vi "DI IRQ Config Pane.vi"(6 "_SubPanelMessages":refnum<notifier>, 9 "_myEmbeddedToFrameEvent":T7, 10 "_myEmbedded.Exit":refnum<user-event>, 11 "_Property Bundle":cluster{"Name":string, "Value":variant}[](array[cluster])) -> (1 "_Connection Informations":T2, 2 "_Scripter Input":T4)   [LabVIEW 2021]
doc: "Registers analog and digital input interrupts and creates timer interrupts."
uses:
  <vilib>/myRIO/Common/Express VI Framework/xctls/myRIO Channel Name/myRIO Channel Name.xctl
  <vilib>/myRIO/Common/Instrument Driver Framework/myRIO v1.0/IRQ/typedefs/DI IRQ Type.ctl
  <vilib>/myRIO/Common/Express VI Framework/typedefs/Config Pane to Framework Ref.ctl
  <vilib>/myRIO/Common/Express VI Framework/typedefs/Data Validate Ref.ctl
  <vilib>/myRIO/Common/Express VI Framework/typedefs/Sub Panel Messages.ctl
  <vilib>/myRIO/Common/Express VI Framework/typedefs/Instrument Driver Method Descriptor Array.ctl
  <vilib>/myRIO/Common/Express VI Framework/typedefs/Instrument Driver Method Descriptor.ctl
  <vilib>/myRIO/Common/Express VI Framework/typedefs/Scripter Input.ctl
  <vilib>/myRIO/Common/Express VI Framework/typedefs/WireThrough Terminal Names.ctl
  <vilib>/myRIO/Common/Express VI Framework/typedefs/Connection Informations.ctl
  <vilib>/myRIO/Common/Instrument Driver Framework/Utilities/typedefs/Channel Types.ctl
  <vilib>/myRIO/Common/Express VI Framework/vis/Express VI Framework Strings Global.vi
  <vilib>/myRIO/Express VI/IRQ/Message Globals.vi
panel:
  out "_create Callback?":bool
  in  "_Create Button":bool
  in  "Callback VI Path:":path
  out "_Warning Icon":picture
  out "_Callback VI Path":string caption="Callback VI:"
  in  "_Open Button":bool
  out "_Count Label":string
  out "_Counts":string[](array[string])=["", "1", "", "1", "", "1", "", "1", "", "1", "", "1"]
  out "_Digtal Preview":T1(graph) caption="Preview:"
  out "_Error Message":string
  in  "_callback":refnum<vi>
  in  "_VI Default Name (Edit and make value default)":string="Digital input interrupt"
  in  "_WireThrough Info (Edit and make value default)":T3={"WireThrough Top In"="Ref In", "WireThrough Bottom In"="error in (no error)", "WireThrough Top Out"="Ref Out", "WireThrough Bottom Out"="error out"}
  in  "_Template Array (Edit and make value default)":T5=[{"Function Name"="Register DI IRQ", "VI Path"=path "<vilib>/myRIO/Instrument Drivers/IRQ/IO IRQ/vis", "Script"=TRUE, "Inputs"=[{"name"="IRQ Number", "value"=variant, "Config Pane Only"=TRUE, "Build Array"=FALSE, "Bundle Cluster"=FALSE, "Show Term"=FALSE, "alias"=[], "Required Input"=FALSE}, {"name"="Digital Interrupt Type", "value"=variant, "Config Pane Only"=TRUE, "Build Array"=FALSE, "Bundle Cluster"=FALSE, "Show Term"=FALSE, "alias"=[], "Required Input"=FALSE}, {"name"="Channel Name", "value"=variant, "Config Pane Only"=TRUE, "Build Array"=FALSE, "Bundle Cluster"=FALSE, "Show Term"=FALSE, "alias"=[], "Required Input"=FALSE}, {"name"="Edge Count", "value"=variant, "Config Pane Only"=TRUE, "Build Array"=FALSE, "Bundle Cluster"=FALSE, "Show Term"=FALSE, "alias"=[], "Required Input"=FALSE}, {"name"="Callback VI Reference", "value"=variant, "Config Pane Only"=FALSE, "Build Array"=FALSE, "Bundle Cluster"=FALSE, "Show Term"=TRUE, "alias"=[], "Required Input"=FALSE}], "Outputs"=[], "VI Class"=enum."Open", "Controls Refs[]"=[], "Inline"=FALSE}]
  in  "_Default Alias String":string
  in  "Type:":T9
  in  "Channel:":u16(xcontrol)
  in  "IRQ number:":u8 max=7
  in  "Edge count:":u32=1 min=1
  in  "Name:":string="Digital input interrupt" caption="Node name:"
  out "_IRQ Learn More":string="Interrupt triggers every time the number of edges reaches the specified Edge count. "
  # "NOTE: Tab Order has been set\nfor this Front Panel.\n\nSee Edit>>Set Tabbing Order...\n\nAll controls that are not visible at \nruntime are excluded from Tabbing order\n\nTo exlude a control from context\nhelp prefix its label text with a '-'"
  # "Trigger point"
  # "Digital input"
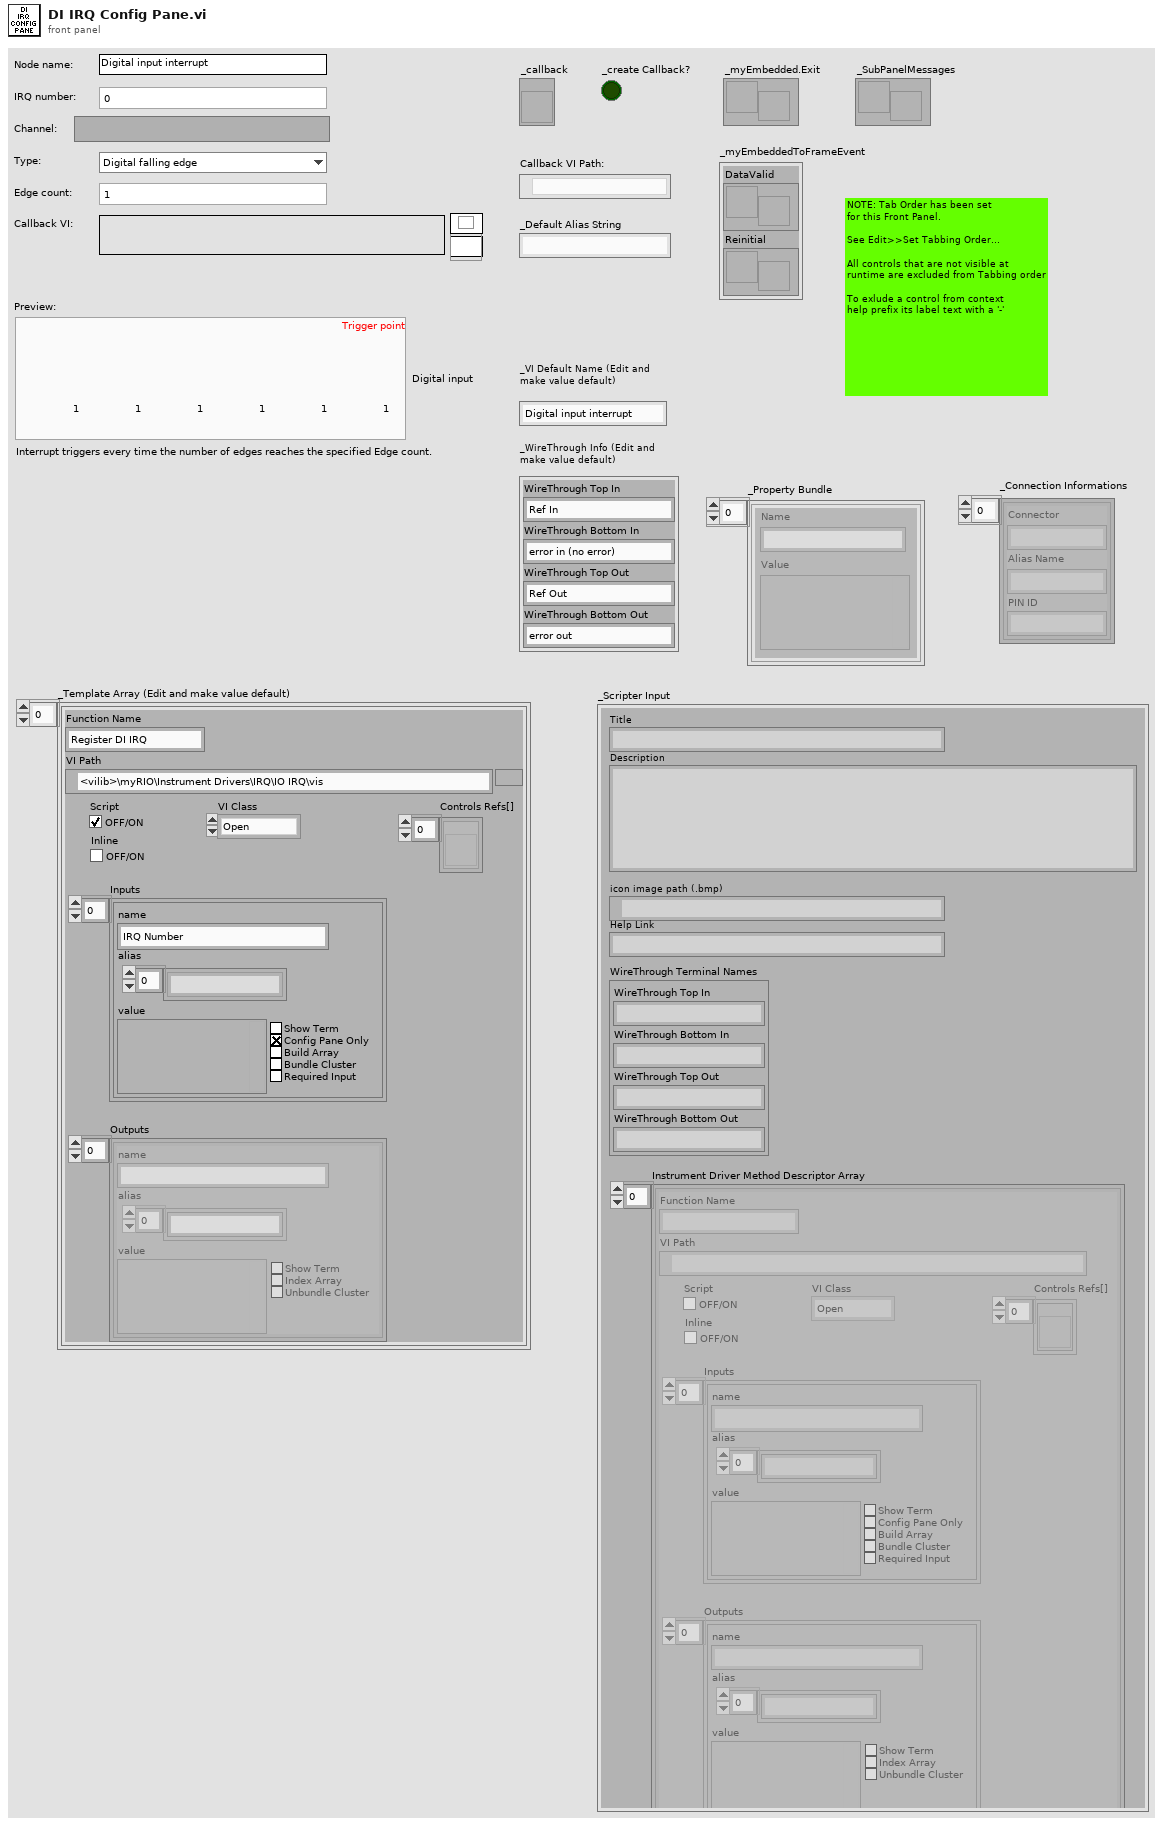
[diagram p1: front panel]
types:
  T1 = cluster{"Analog Preview 3":cluster{"X":dbl, "Y":dbl}[]}[]
  T2 = typedef "Connection Informations.ctl" = cluster{"Connector":string, "Alias Name":string, "PIN ID":string}[]
  T3 = typedef "WireThrough Terminal Names.ctl" = cluster{"WireThrough Top In":string, "WireThrough Bottom In":string, "WireThrough Top Out":string, "WireThrough Bottom Out":string}
  T4 = typedef "Scripter Input.ctl" = cluster{"Title":string, "Description":string, "icon image path (.bmp)":path, "Help Link":string, "WireThrough Terminal Names":T3, "Instrument Driver Method Descriptor Array":T5}
  T5 = typedef "Instrument Driver Method Descriptor Array.ctl" = T6[]
  T6 = typedef "Instrument Driver Method Descriptor.ctl" = cluster{"Function Name":string, "VI Path":path, "Script":bool, "Inputs":cluster{"name":string, "value":variant, "Config Pane Only":bool, "Build Array":bool, "Bundle Cluster":bool, "Show Term":bool, "alias":string[], "Required Input":bool}[], "Outputs":cluster{"name":string, "value":variant, "Show Term":bool, "Index Array":bool, "Unbundle Cluster":bool, "alias":string[]}[], "VI Class":enum16{"Open", "Configure", "Data", "Manage", "Close"}, "Controls Refs[]":refnum<vi>[], "Inline":bool}
  T7 = typedef "Config Pane to Framework Ref.ctl" = cluster{"DataValid":T8, "Reinitial":refnum<user-event>}
  T8 = typedef "Data Validate Ref.ctl" = refnum<user-event>
  T9 = typedef "DI IRQ Type.ctl" = enum16{"Digital falling edge", "Digital rising edge", "Digital edge"}
  T10 = typedef "Channel Types.ctl" = enum32{"Unknown", "AI", "AO", "DIO - DI", "DIO", "DIO - DO", "I2C", "PWM", "Encoder", "SPI", "UART", "Accelerometer", "DIO - LED", "DIO - Button", "AI (N Samples)", "AudioIn (N Samples)", "AO (N Samples)", "AudioOut (N Samples)", "DI (N Samples)", "DO (N Samples)", "AI IRQ", "DI IRQ", "Timer IRQ", "RSL", "Relay", "CAN", "AI (Continuous)", "AO (Continuous)"}
  T11 = typedef "Channel Info.ctl" = cluster{"Channel Name":string, "Alias":string, "Used?":bool, "Not Support?":bool, "Property Bundle":cluster{"Name":string, "Value":variant}[]}
  T12 = typedef "Sub Panel Messages.ctl" = enum16{"Initialized"}
  T13 = cluster{"Connector":string, "Alias Name":string, "PIN ID":string}
  T14 = cluster{"left":i16, "top":i16, "right":i16, "bottom":i16}
  T15 = cluster{"name":string, "value":variant, "Config Pane Only":bool, "Build Array":bool, "Bundle Cluster":bool, "Show Term":bool, "alias":string[], "Required Input":bool}[]
  T16 = cluster{"name":string, "value":variant, "Config Pane Only":bool, "Build Array":bool, "Bundle Cluster":bool, "Show Term":bool, "alias":string[], "Required Input":bool}
  T17 = cluster{"Connector":string, "Alias Name":string, "PIN ID":string}[]
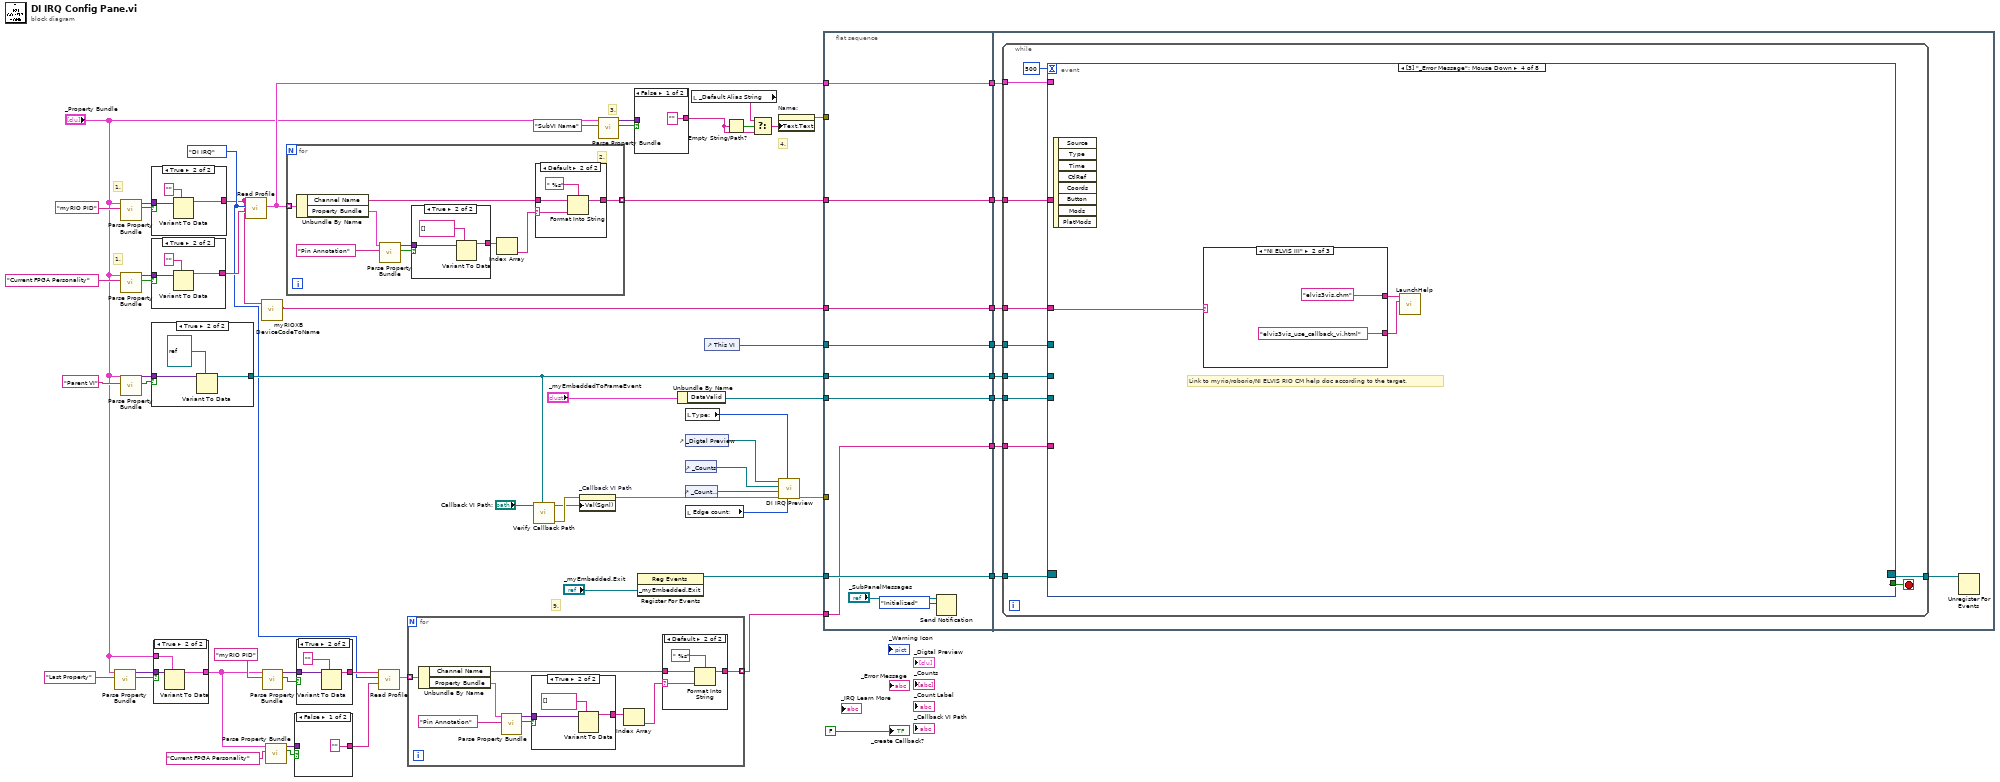
[diagram p0: block diagram]
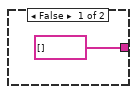
[diagram p2: hidden frame]
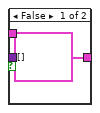
[diagram p4: hidden frame]
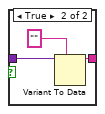
[diagram p5: hidden frame]
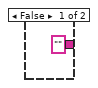
[diagram p6: hidden frame]
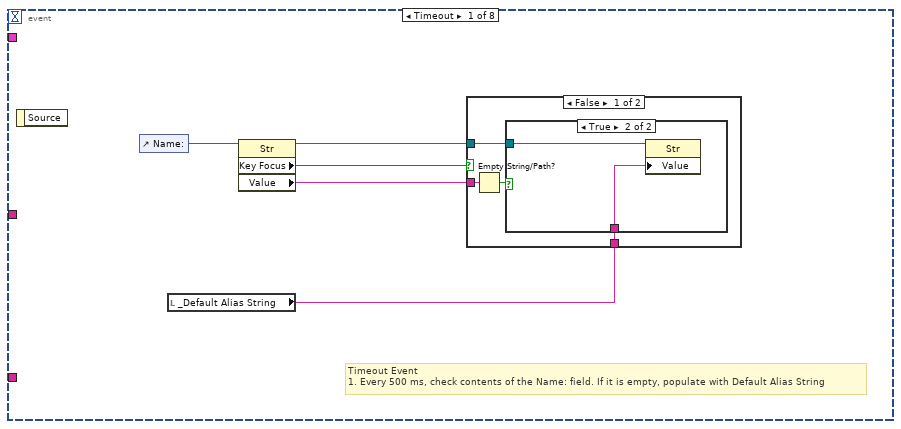
[diagram p7: hidden frame]
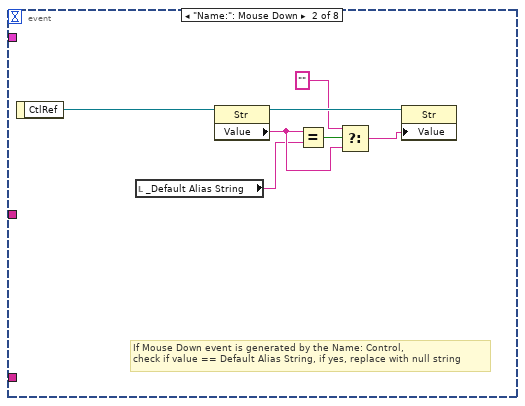
[diagram p10: hidden frame]
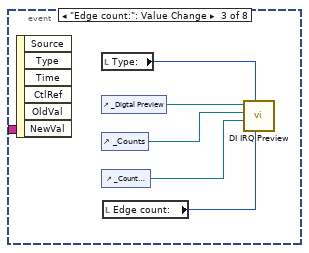
[diagram p11: hidden frame]
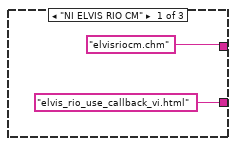
[diagram p12: hidden frame]
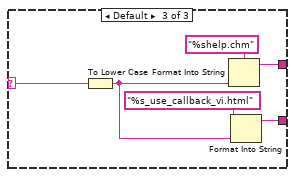
[diagram p13: hidden frame]
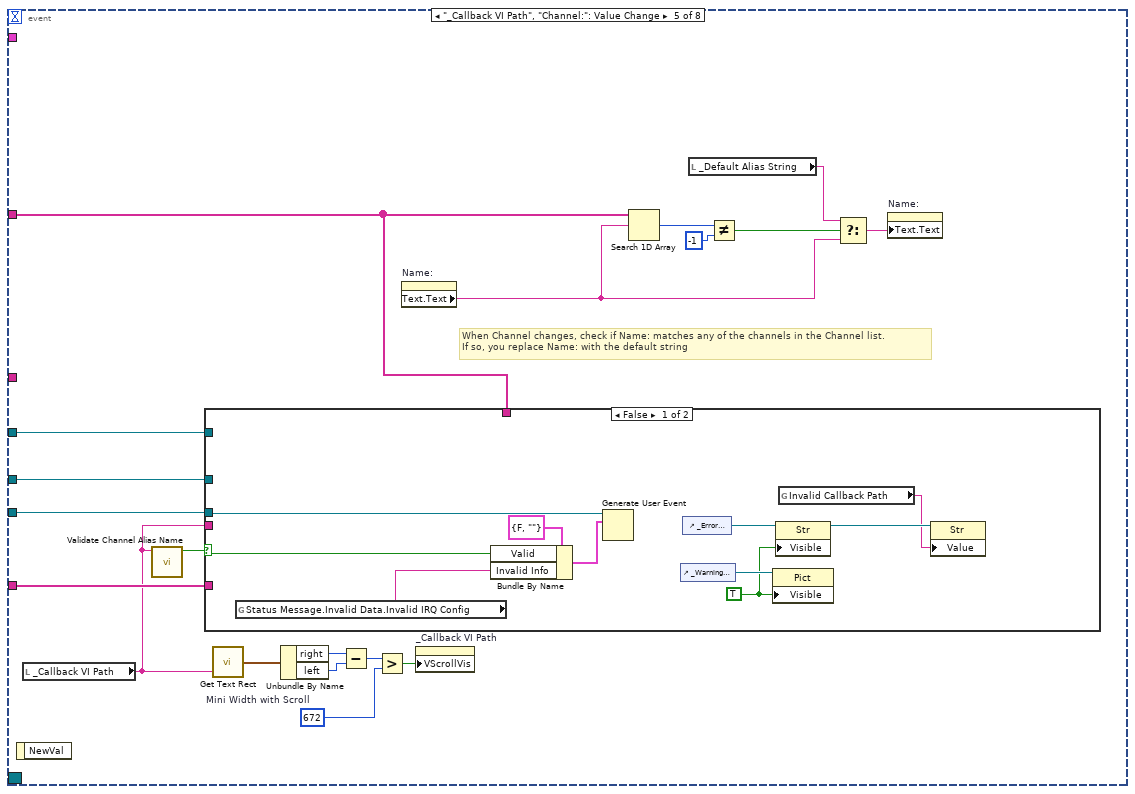
[diagram p14: hidden frame]
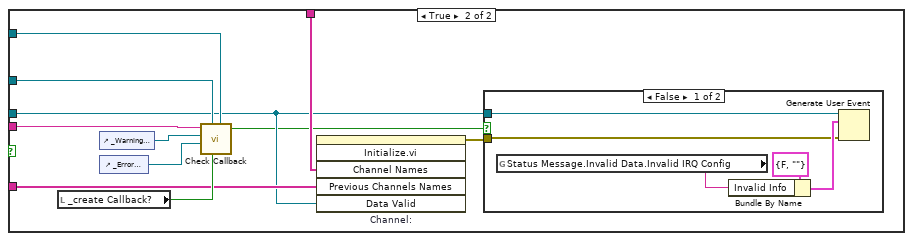
[diagram p15: hidden frame]
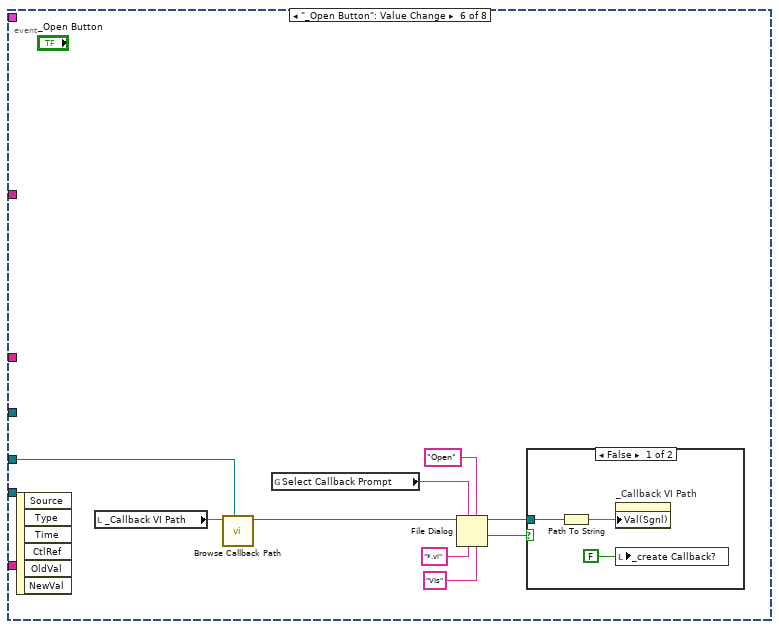
[diagram p17: hidden frame]
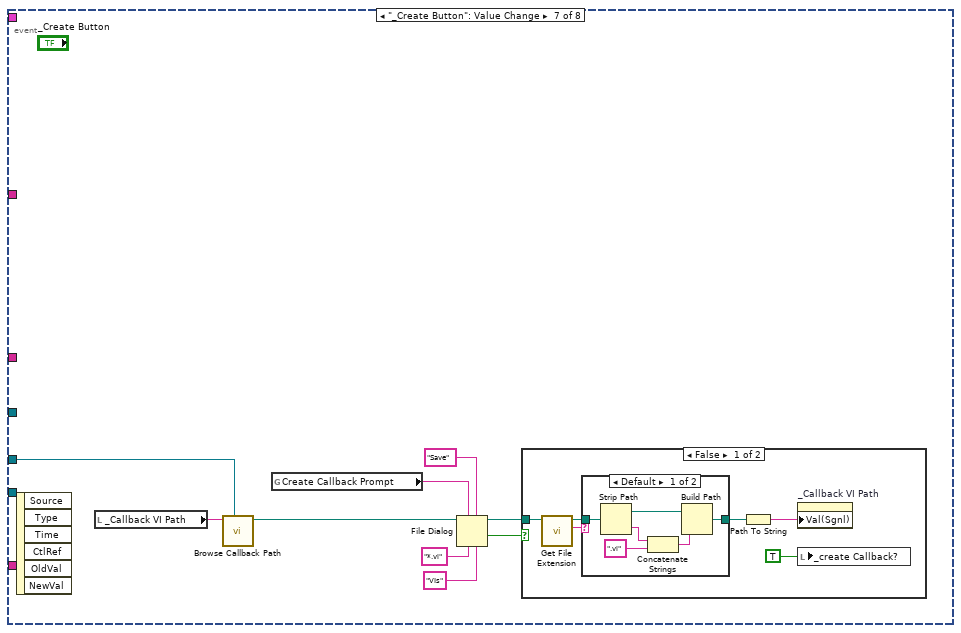
[diagram p19: hidden frame]
diagram:
  w6 = Channel_Types."DI IRQ" ("Channel to Read")
  # "1."
  # "1."
  # "9."
  # "4."
  # "3."
  n1 = call <vilib>:"Parse Property Bundle.vi"("Name"="Last Property", "Property Bundle"="_Property Bundle") -> ("Found?"=w10:bool, "Value"=w11:variant)  [unwired: 8 in]
  n2 = call <vilib>:"Parse Property Bundle.vi"("Name"="myRIO PID", "Property Bundle"="_Property Bundle") -> ("Found?"=w53:bool, "Value"=w54:variant)  [unwired: 8 in]
  n3 = call <vilib>:"Parse Property Bundle.vi"("Name"="Current FPGA Personality", "Property Bundle"="_Property Bundle") -> ("Found?"=w52:bool, "Value"=w51:variant)  [unwired: 8 in]
  n4 = call <vilib>:"Parse Property Bundle.vi"("Name"="Parent VI", "Property Bundle"="_Property Bundle") -> ("Found?"=w44:bool, "Value"=w45:variant)  [unwired: 8 in]
  n5 = case shown="True" w53 {
    tunnel: w54 -> [_ w67]
    tunnel: ["" ("Name") w65] -> w2
    frame False {
    }
    frame True {
      n6 = Variant To Data(type="" ("Name"), Variant=w67) -> (data=w65:string)  [unwired: 1 in, 1 out]
    }
  }
  n7 = case shown="True" w52 {
    tunnel: w51 -> [_ w71]
    tunnel: ["" ("Name") w69] -> w49
    frame False {
    }
    frame True {
      n8 = Variant To Data(type="" ("Name"), Variant=w71) -> (data=w69:string)  [unwired: 1 in, 1 out]
    }
  }
  n9 = case shown="True" w44 {
    tunnel: w45 -> [_ w75]
    tunnel: [refnum<vi> refnum ("reference out") w73] -> w38
    frame False {
    }
    frame True {
      n10 = Variant To Data(type=refnum<vi> refnum ("reference out"), Variant=w75) -> (data=w73:refnum<vi>)  [unwired: 1 in, 1 out]
    }
  }
  n11 = case shown="True" w10 {
    tunnel: w11 -> [_ w79]
    tunnel: [cluster{"Name":string, "Value":variant}[] [] ("_Property Bundle") w78] -> w9
    tunnel: "_Property Bundle" -> [_ w77]
    frame False {
    }
    frame True {
      n12 = Variant To Data(type=w77, Variant=w79) -> (data=w78:cluster{"Name":string, "Value":variant}[])  [unwired: 1 in, 1 out]
    }
  }
  n13 = call <vilib>:"Read Profile.vi"("FPGA Name"=w49, "Channel to Read"=w6, "myRIO PID"=w2) -> ("Channel List Out"=w47:T11[])  [unwired: 7 in, 1 out]
  n14 = call <vilib>:"myRIOXB DeviceCodeToName.vi"("Device Code"=w2) -> ("Name"=w1:string)  [unwired: 10 in]
  n15 = call <vilib>:"Parse Property Bundle.vi"("Name"="myRIO PID", "Property Bundle"=w9) -> ("Found?"=w19:bool, "Value"=w18:variant)  [unwired: 8 in]
  n16 = call <vilib>:"Parse Property Bundle.vi"("Name"="Current FPGA Personality", "Property Bundle"=w9) -> ("Found?"=w14:bool, "Value"=w15:variant)  [unwired: 8 in]
  n17 = for {
    tunnel: w47 -> [w87] mode=indexing
    tunnel: [w88] -> w22 mode=indexing
    # "2."
    n18 = Unbundle By Name(w87) -> ("Channel Name"=w86:string, "Property Bundle"=w85:cluster{"Name":string, "Value":variant}[])
    n19 = call <vilib>:"Parse Property Bundle.vi"("Name"="Pin Annotation", "Property Bundle"=w85) -> ("Found?"=w82:bool, "Value"=w83:variant)  [unwired: 8 in]
    n20 = case shown="True" w82 {
      tunnel: w83 -> [_ w92]
      tunnel: [string[] [] w91] -> w81
      frame False {
      }
      frame True {
        n21 = Variant To Data(type=string[] [], Variant=w92) -> (data=w91:string[])  [unwired: 1 in, 1 out]
      }
    }
    n22 = Index Array(array=w81) -> (element=w80:string)  [unwired: 1 in]
    n23 = case shown="Default" w80 {
      selector: w80 -> [_ w96]
      tunnel: w86 -> [w93 w95]
      tunnel: [w93 w94] -> w88
      frame "" {
      }
      frame Default {
        n24 = Format Into String(format string=" %s", initial string=w95, w96) -> (resulting string=w94:string)  [unwired: 1 in, 1 out]
      }
    }
  }
  n25 = case shown="False" w14 {
    tunnel: w15 -> [_ w101]
    tunnel: ["" ("Name") w99] -> w13
    frame False {
    }
    frame True {
      n26 = Variant To Data(type="" ("Name"), Variant=w101) -> (data=w99:string)  [unwired: 1 in, 1 out]
    }
  }
  n27 = case shown="True" w19 {
    tunnel: w18 -> [_ w105]
    tunnel: ["" ("Name") w103] -> w20
    frame False {
    }
    frame True {
      n28 = Variant To Data(type="" ("Name"), Variant=w105) -> (data=w103:string)  [unwired: 1 in, 1 out]
    }
  }
  n29 = call <vilib>:"Read Profile.vi"("FPGA Name"=w13, "Channel to Read"=w6, "myRIO PID"=w20) -> ("Channel List Out"=w8:T11[])  [unwired: 7 in, 1 out]
  n30 = for {
    tunnel: w8 -> [w113] mode=indexing
    tunnel: [w114] -> w5 mode=indexing
    n31 = Unbundle By Name(w113) -> ("Channel Name"=w112:string, "Property Bundle"=w111:cluster{"Name":string, "Value":variant}[])
    n32 = call <vilib>:"Parse Property Bundle.vi"("Name"="Pin Annotation", "Property Bundle"=w111) -> ("Found?"=w108:bool, "Value"=w109:variant)  [unwired: 8 in]
    n33 = case shown="True" w108 {
      tunnel: w109 -> [_ w118]
      tunnel: [string[] [] w117] -> w107
      frame False {
      }
      frame True {
        n34 = Variant To Data(type=string[] [], Variant=w118) -> (data=w117:string[])  [unwired: 1 in, 1 out]
      }
    }
    n35 = Index Array(array=w107) -> (element=w106:string)  [unwired: 1 in]
    n36 = case shown="Default" w106 {
      selector: w106 -> [_ w122]
      tunnel: w112 -> [w119 w121]
      tunnel: [w119 w120] -> w114
      frame "" {
      }
      frame Default {
        n37 = Format Into String(format string=" %s", initial string=w121, w122) -> (resulting string=w120:string)  [unwired: 1 in, 1 out]
      }
    }
  }
  n38 = call <vilib>:"Verify Callback Path.vi"("Parent VI Ref"=w38, "Saved Callback Path"="Callback VI Path:") -> ("error out"=w37:errorcluster, "Valid Path out"=w36:string)  [unwired: 8 in]
  n39 = property on="_Callback VI Path" class="Str"(error in=w37, "Val(Sgnl)"=w36) -> (error out=w35:errorcluster)  [unwired: 1 in, 1 out]
  n40 = call <vilib>:"Parse Property Bundle.vi"("Name"="SubVI Name", "Property Bundle"="_Property Bundle") -> ("Found?"=w58:bool, "Value"=w57:variant)  [unwired: 8 in]
  n41 = case shown="False" w58 {
    tunnel: w57 -> [_ w127]
    tunnel: ["" ("Name") w125] -> w56
    frame False {
    }
    frame True {
      n42 = Variant To Data(type="" ("Name"), Variant=w127) -> (data=w125:string)  [unwired: 1 in, 1 out]
    }
  }
  n43 = register-events("_myEmbedded.Exit") -> (reference out=w48:refnum<event-registration>)  [unwired: 2 in, 1 out]
  n44 = Unbundle By Name("_myEmbeddedToFrameEvent") -> ("DataValid"=w30:T8)
  n45 = local read "Type:"() -> (w42:T9)
  n46 = control-ref of="_Digtal Preview"() -> (w39:refnum<vi>)
  n47 = control-ref of="_Counts"() -> (w40:refnum<vi>)
  n48 = control-ref of="_Count Label"() -> (w41:refnum<vi>)
  n49 = local read "Edge count:"() -> (w43:u32)
  n50 = local read "_Default Alias String"() -> (w60:string)
  n51 = control-ref of="This VI"() -> (w34:refnum<vi>)
  n52 = Empty String/Path?(string/path=w56) -> (empty?=w62:bool)
  n53 = Select(t=w60, s=w62, f=w56) -> (s? t:f=w61:string)
  n54 = property on="Name:" class="Str"("Text.Text"=w61) -> (error out=w3:errorcluster)  [unwired: 2 in, 1 out]
  n55 = call <vilib>:"DI IRQ Preview.vi"("Edge Count:"=w43, "Type:"=w42, "error in (no error)"=w35, "_Count Label Refnum"=w41, "_Counts Refnum"=w40, "_Digtal Preview Refnum"=w39) -> ("error out"=w32:errorcluster)  [unwired: 5 in]
  n56 = flat-sequence {
    tunnel: w30 -> [w130]
    tunnel: w32 -> [_]
    tunnel: w34 -> [w134]
    tunnel: w38 -> [w135]
    tunnel: w47 -> [w136]
    tunnel: w48 -> [w137]
    tunnel: [w137] -> w29
    tunnel: [w136] -> w28
    tunnel: [w135] -> w27
    tunnel: [w134] -> w26
    tunnel: [w130] -> w25
    tunnel: [w131] -> w23
    tunnel: w1 -> [w131]
    tunnel: w22 -> [w129]
    tunnel: [w129] -> w21
    tunnel: w5 -> [w128]
    tunnel: [w128] -> w4
    tunnel: w3 -> [_]
    tunnel: w29 -> [w146]
    tunnel: w28 -> [w145]
    tunnel: w27 -> [w143]
    tunnel: w26 -> [w142]
    tunnel: w25 -> [w141]
    tunnel: w23 -> [w140]
    tunnel: w21 -> [w139]
    tunnel: w4 -> [w138]
    frame #0 {
      n57 = Send Notification(notification=Sub_Panel_Messages."Initialized", notifier="_SubPanelMessages") -> ()  [unwired: 1 in, 2 out]
    }
    frame #1 {
      n58 = while {
        tunnel: w146 -> [w156]
        tunnel: w141 -> [w152]
        tunnel: w145 -> [w153]
        tunnel: [w154] -> w144
        tunnel: w143 -> [w151]
        tunnel: w142 -> [w150]
        tunnel: w140 -> [w149]
        tunnel: w139 -> [w148]
        tunnel: w138 -> [w147]
        stop <- w155 stop-if-true
        n59 = event shown="[3] \"_Error Message\": Mouse Down" {
          selector: w156 -> [_ _ _ _ _ _ _ _]
          dyn-events: [_ _ _ _ _ _ _ _] -> w154
          timeout: 500 -> [_ _ _ _ _ _ _ _]
          tunnel: [_ _ _ _ _ _ _ TRUE ("Valid Callback?")] -> w155
          tunnel: w153 -> [_ _ _ _ _ _ _ w304]
          tunnel: w152 -> [_ _ _ _ w196 _ _ _]
          tunnel: w151 -> [_ _ _ _ w212 w239 w252 w278]
          tunnel: w150 -> [_ _ _ _ w211 _ _ _]
          tunnel: w149 -> [_ _ _ w181 _ _ _ _]
          tunnel: w148 -> [_ _ _ _ w198 _ _ _]
          tunnel: w147 -> [_ _ _ _ w197 _ _ _]
          event Timeout {
            # "Timeout Event\n1. Every 500 ms, check contents of the Name: field. If it is empty, populate with Default Alias String"
            n60 = event-data() -> ()  [unwired: 1 in, 1 out]
            n61 = control-ref of="Name:"() -> (w159:refnum<vi>)
            n62 = local read "_Default Alias String"() -> (w158:string)
            n63 = property on="Property Node" class="Str"(reference=w159) -> (reference out=w162:refnum<vi>, "Key Focus"=w161:bool, "Value"=w160:string)  [unwired: 1 in, 1 out]
            n64 = case shown="False" w161 {
              tunnel: w160 -> [w166 _]
              tunnel: w162 -> [w164 _]
              tunnel: w158 -> [w163 _]
              frame False {
                n65 = Empty String/Path?(string/path=w166) -> (empty?=w165:bool)
                n66 = case shown="True" w165 {
                  tunnel: w164 -> [_ w168]
                  tunnel: w163 -> [_ w167]
                  frame False {
                  }
                  frame True {
                    n67 = property on="Property Node" class="Str"(reference=w168, "Value"=w167) -> ()  [unwired: 1 in, 2 out]
                  }
                }
              }
              frame True {
              }
            }
          }
          event "Name:": Mouse Down {
            # "If Mouse Down event is generated by the Name: Control,\ncheck if value == Default Alias String, if yes, replace with null string"
            n68 = event-data() -> ("CtlRef"=w170:refnum<vi>)  [unwired: 1 in]
            n69 = local read "_Default Alias String"() -> (w169:string)
            n70 = property class="Str"(reference=w170) -> (reference out=w174:refnum<vi>, "Value"=w175:string)  [unwired: 1 in, 1 out]
            n71 = Equal?(x=w175, y=w169) -> (x = y?=w171:bool)
            n72 = Select(t="", s=w171, f=w175) -> (s? t:f=w173:string)
            n73 = property class="Str"(reference=w174, "Value"=w173) -> ()  [unwired: 1 in, 2 out]
          }
          event "Edge count:": Value Change {
            n74 = event-data() -> ()  [unwired: 1 in, 6 out]
            n75 = local read "Type:"() -> (w177:T9)
            n76 = control-ref of="_Digtal Preview"() -> (w180:refnum<vi>)
            n77 = control-ref of="_Counts"() -> (w179:refnum<vi>)
            n78 = control-ref of="_Count Label"() -> (w178:refnum<vi>)
            n79 = local read "Edge count:"() -> (w176:u32)
            n80 = call <vilib>:"DI IRQ Preview.vi"("Edge Count:"=w176, "Type:"=w177, "_Count Label Refnum"=w178, "_Counts Refnum"=w179, "_Digtal Preview Refnum"=w180) -> ()  [unwired: 6 in, 1 out]
          }
          event "_Error Message": Mouse Down {
            # "Link to myrio/roborio/NI ELVIS RIO CM help doc according to the target."
            n81 = event-data() -> ()  [unwired: 1 in, 8 out]
            n82 = case shown="\"NI ELVIS III\"" w181 {
              selector: w181 -> [_ _ w188]
              tunnel: ["elvisriocm.chm" ("Help File") "elvis3vis.chm" ("Help File") w190] -> w183
              tunnel: ["elvis_rio_use_callback_vi.html" ("Help Topic") "elvis3vis_use_callback_vi.html" ("Help Topic") w189] -> w182
              frame "NI ELVIS RIO CM" {
              }
              frame "NI ELVIS III" {
              }
              frame Default {
                n83 = To Lower Case(string=w188) -> (all lower case string=w192:string)
                n84 = Format Into String(format string="%shelp.chm" ("Help File"), w192) -> (resulting string=w190:string)  [unwired: 2 in, 1 out]
                n85 = Format Into String(format string="%s_use_callback_vi.html" ("Help Topic"), w192) -> (resulting string=w189:string)  [unwired: 2 in, 1 out]
              }
            }
            n86 = call <vilib>:"LaunchHelp.vi"("Help Topic"=w182, "Help File"=w183) -> ()  [unwired: 10 in]
          }
          event "_Callback VI Path", "Channel:": Value Change {
            w206 = i16 672  # Mini Width with Scroll
            # "When Channel changes, check if Name: matches any of the channels in the Channel list. \nIf so, you replace Name: with the default string"
            n87 = event-data() -> ()  [unwired: 1 in, 1 out]
            n88 = local read "_Callback VI Path"() -> (w194:string)
            n89 = call <vilib>:"Validate Channel Alias Name.vi"("Channel Alias"=w194) -> ("Valid?"=w195:bool)  [unwired: 9 in, 1 out]
            n90 = case shown="False" w195 {
              selector: w195 -> [w219 _]
              tunnel: w212 -> [_ w233]
              tunnel: w211 -> [_ w230]
              tunnel: w194 -> [_ w228]
              tunnel: w198 -> [_ w227]
              tunnel: w197 -> [_ w226]
              tunnel: w196 -> [w220 w225]
              frame False {
                w216 = TRUE ("Visible")
                n91 = global read "Express VI Framework Strings Global.vi" "Status Message.Invalid Data.Invalid IRQ Config"() -> (w215:string)
                n92 = Bundle By Name(cluster=cluster{"Valid":bool, "Invalid Info":string} {"Valid"=FALSE, "Invalid Info"=""} ("event data"), "Valid"=w219, "Invalid Info"=w215) -> (w221:cluster{"Valid":bool, "Invalid Info":string})
                n93 = Generate User Event(user event=w220, event data cluster=w221) -> ()  [unwired: 2 in, 2 out]
                n94 = control-ref of="_Warning Icon"() -> (w217:refnum<vi>)
                n95 = control-ref of="_Error Message"() -> (w218:refnum<vi>)
                n96 = property class="Pict"(reference=w217, "Visible"=w216) -> ()  [unwired: 1 in, 2 out]
                n97 = property class="Str"(reference=w218, "Visible"=w216) -> (reference out=w214:refnum<vi>)  [unwired: 1 in, 1 out]
                n98 = global read "Message Globals.vi" "Invalid Callback Path"() -> (w213:string)
                n99 = property class="Str"(reference=w214, "Value"=w213) -> ()  [unwired: 1 in, 2 out]
              }
              frame True {
                n100 = local read "_create Callback?"() -> (w229:bool)
                n101 = control-ref of="_Warning Icon"() -> (w232:refnum<vi>)
                n102 = control-ref of="_Error Message"() -> (w231:refnum<vi>)
                n103 = call <vilib>:"Check Callback.vi"("Config VI Ref"=w230, "Create Callback?"=w229, "Parent VI Ref"=w233, "Error Message Ref"=w231, "Warning Icon Ref"=w232, "Callback Path"=w228) -> ("Valid Callback?"=w223:bool)  [unwired: 5 in]
                n104 = invoke on="Channel:" class="myRIO Channel Name (strict)" method="Initialize.vi"("Channel Names"=w227, "Previous Channels Names"=w226, "Data Valid"=w225) -> (error out=w224:errorcluster)  [unwired: 3 in, 5 out]
                n105 = case shown="False" w223 {
                  tunnel: w225 -> [w236 _]
                  tunnel: w224 -> [w234 _]
                  frame False {
                    n106 = global read "Express VI Framework Strings Global.vi" "Status Message.Invalid Data.Invalid IRQ Config"() -> (w235:string)
                    n107 = Bundle By Name(cluster=cluster{"Valid":bool, "Invalid Info":string} {"Valid"=FALSE, "Invalid Info"=""} ("event data"), "Invalid Info"=w235) -> (w238:cluster{"Valid":bool, "Invalid Info":string})
                    n108 = Generate User Event(user event=w236, event data cluster=w238, error in=w234) -> ()  [unwired: 1 in, 2 out]
                  }
                  frame True {
                  }
                }
              }
            }
            n109 = call <vilib>:"Get Text Rect.vi"("text"=w194) -> ("rect"=w210:T14)  [unwired: 8 in]
            n110 = Unbundle By Name(w210) -> ("right"=w209:i16, "left"=w208:i16)
            n111 = Subtract(x=w209, y=w208) -> (x-y=w207:i16)
            n112 = Greater?(x=w207, y=w206) -> (0:w205:bool)
            n113 = property on="Name:" class="Str"() -> ("Text.Text"=w200:string)  [unwired: 2 in, 2 out]
            n114 = property on="_Callback VI Path" class="Str"("VScrollVis"=w205) -> ()  [unwired: 2 in, 2 out]
            n115 = Search 1D Array(1D array=w198, element=w200) -> (index of element=w203:i32)  [unwired: 1 in]
            n116 = local read "_Default Alias String"() -> (w202:string)
            n117 = Not Equal?(x=w203, y=-1) -> (x != y?=w204:bool)
            n118 = Select(t=w202, s=w204, f=w200) -> (s? t:f=w201:string)
            n119 = property on="Name:" class="Str"("Text.Text"=w201) -> ()  [unwired: 2 in, 2 out]
          }
          event "_Open Button": Value Change {
            n120 = event-data() -> ()  [unwired: 1 in, 6 out]
            n121 = local read "_Callback VI Path"() -> (w241:string)
            n122 = call <vilib>:"Browse Callback Path.vi"("Parent VI Ref"=w239, "Init Path in"=w241) -> ("Init Path out"=w240:path)  [unwired: 9 in]
            n123 = global read "Message Globals.vi" "Select Callback Prompt"() -> (w243:string)
            n124 = File Dialog(4:"VIs" ("pattern label"), 5:"Open" ("button label"), 6:"*.vi" ("pattern (all files)"), 7:w243, 11:w240) -> (1:w245:bool, 3:w244:path)  [unwired: 2 in, 2 out]
            n125 = case shown="False" w245 {
              tunnel: w244 -> [w250 _]
              frame False {
                n126 = Path To String(path=w250) -> (string=w249:string)
                n127 = property on="_Callback VI Path" class="Str"("Val(Sgnl)"=w249) -> ()  [unwired: 2 in, 2 out]
                n128 = local write "_create Callback?"(FALSE ("_create Callback?")) -> ()
              }
              frame True {
              }
            }
          }
          event "_Create Button": Value Change {
            n129 = event-data() -> ()  [unwired: 1 in, 6 out]
            n130 = local read "_Callback VI Path"() -> (w253:string)
            n131 = call <vilib>:"Browse Callback Path.vi"("Parent VI Ref"=w252, "Init Path in"=w253) -> ("Init Path out"=w251:path)  [unwired: 9 in]
            n132 = global read "Message Globals.vi" "Create Callback Prompt"() -> (w255:string)
            n133 = File Dialog(4:"VIs" ("pattern label"), 5:"Save" ("button label"), 6:"*.vi" ("pattern (all files)"), 7:w255, 11:w251) -> (1:w257:bool, 3:w256:path)  [unwired: 2 in, 2 out]
            n134 = case shown="False" w257 {
              tunnel: w256 -> [w261 _]
              frame False {
                n135 = call <vilib>:"Get File Extension.vi"("file"=w261) -> ("lowercase file extension"=w262:string, "dup file"=w263:path)  [unwired: 6 in, 3 out]
                n136 = case shown="Default" w262 {
                  tunnel: w263 -> [w271 w272]
                  tunnel: [w267 w272] -> w260
                  frame Default {
                    n137 = Strip Path(path=w271) -> (stripped path=w270:path, name=w269:string)
                    n138 = Concatenate Strings(w269, ".vi" ("string")) -> (w268:string)
                    n139 = Build Path(base path=w270, name or relative path=w268) -> (appended path=w267:path)
                  }
                  frame "vi" {
                  }
                }
                n140 = Path To String(path=w260) -> (string=w265:string)
                n141 = property on="_Callback VI Path" class="Str"("Val(Sgnl)"=w265) -> ()  [unwired: 2 in, 2 out]
                n142 = local write "_create Callback?"(TRUE ("_create Callback?")) -> ()
              }
              frame True {
              }
            }
          }
          event User Event {
            w288 = 0
            n143 = event-data() -> ("myEmbedded.Exit"=w274:bool)  [unwired: 1 in]
            n144 = property on="_Callback VI Path" class="Str"() -> ("Value"=w275:string)  [unwired: 2 in, 2 out]
            n145 = case shown="False" w274 {
              tunnel: w278 -> [_ w330]
              tunnel: [w324 w328] -> w276
              tunnel: w275 -> [w324 w327]
              frame False {
              }
              frame True {
                n146 = local read "_create Callback?"() -> (w326:bool)
                n147 = vi-ref <vilib>:"IO IRQ Callback .vit"() -> (w325:refnum<vi>)
                n148 = call <vilib>:"Create Callback.vi"("Create Callback?"=w326, "Parent VI Ref"=w330, "Template VI Ref"=w325, "Callback Path"=w327) -> ("Saved Callback Path"=w329:path, "Dup Callback Path"=w328:string)  [unwired: 6 in]
                n149 = local write "Callback VI Path:"(w329) -> ()
              }
            }
            n150 = Index Array(array=w304, index="Channel:") -> (element=w305:T11)
            n151 = Unbundle By Name(w305) -> ("Channel Name"=w281:string, "Property Bundle"=w279:cluster{"Name":string, "Value":variant}[])
            n152 = Build Array(w276) -> (w287:string[])
            n153 = in-place {
              in-place-border: "IRQ number:" -> [w338]
              in-place-border: "Type:" -> [w337]
              in-place-border: w281 -> [w336]
              in-place-border: "Edge count:" -> [w335]
              in-place-border: "_callback" -> [w334]
              in-place-border: w288 -> [w332]
              in-place-border: w287 -> [w331]
              n154 = in-place-array #1("_Template Array (Edit and make value default)", w288) -> (w339:T6)
              n155 = in-place {
                in-place-border: w338 -> [w351]
                in-place-border: w337 -> [w350]
                in-place-border: w336 -> [w349]
                in-place-border: w335 -> [w348]
                in-place-border: w334 -> [w347]
                in-place-border: w332 -> [w340]
                in-place-border: w331 -> [w341]
                n156 = in-place-cluster #2(w339) -> ("Inputs"=w352:T15)
                n157 = in-place {
                  in-place-border: w351 -> [w365]
                  in-place-border: w350 -> [w364]
                  in-place-border: w349 -> [w363]
                  in-place-border: w348 -> [w362]
                  in-place-border: w347 -> [w361]
                  in-place-border: w341 -> [w353]
                  n158 = in-place-array #3(w352, w340, 1, 2, 3, 4) -> (w368:T16, w367:T16, w366:T16, w360:T16, w359:T16)
                  n159 = Bundle By Name(cluster=w368, "value"=w365) -> (w354:T16)
                  n160 = Bundle By Name(cluster=w367, "value"=w364) -> (w355:T16)
                  n161 = Bundle By Name(cluster=w366, "value"=w363) -> (w356:T16)
                  n162 = Bundle By Name(cluster=w360, "value"=w362) -> (w357:T16)
                  n163 = Bundle By Name(cluster=w359, "value"=w361, "alias"=w353) -> (w358:T16)
                  n164 = in-place-array #3(w354, w355, w356, w357, w358) -> (w346:T15)  [unwired: 5 out]
                }
                n165 = in-place-cluster #2("Inputs"=w346) -> (w333:T6)
              }
              n166 = in-place-array #1(w333) -> (w294:T5)  [unwired: 1 out]
            }
            n167 = Match Pattern(string=w281, regular expression="/") -> (before substring=w284:string, after substring=w285:string, offset past match=w273:i32)  [unwired: 1 in, 1 out]
            n168 = case shown="Default" w273 {
              tunnel: w285 -> [_ w322]
              tunnel: w284 -> [_ w320]
              tunnel: [T13 {"Connector"="Onboard", "Alias Name"="Button0", "PIN ID"=""} ("Connection Information") w319] -> w282
              tunnel: w279 -> [_ w314]
              frame -1 {
              }
              frame Default {
                n169 = call <vilib>:"Parse Property Bundle.vi"("Name"="Pin Annotation" ("x"), "Property Bundle"=w314) -> ("Value"=w315:variant)  [unwired: 8 in, 1 out]
                n170 = Variant To Data(type=string[] [], Variant=w315) -> (data=w317:string[])  [unwired: 1 in, 1 out]
                n171 = Concatenate Strings("Connector " ("string"), w320) -> (w321:string)
                n172 = call <vilib>:"Trim Whitespace.vi"("string"=w322) -> ("trimmed string"=w323:string)  [unwired: 1 in]
                n173 = Index Array(array=w317) -> (element=w308:string)  [unwired: 1 in]
                n174 = Match Pattern(string=w308, regular expression="(") -> (after substring=w310:string)  [unwired: 1 in, 3 out]
                n175 = Match Pattern(string=w310, regular expression=")") -> (before substring=w307:string)  [unwired: 1 in, 3 out]
                n176 = Bundle By Name(cluster=T13 {"Connector"="", "Alias Name"="", "PIN ID"=""} ("Connection Information"), "Connector"=w321, "Alias Name"=w323, "PIN ID"=w307) -> (w319:T13)
              }
            }
            n177 = Equal?(x="_Default Alias String", y="Name:") -> (x = y?=w297:bool)
            n178 = Select(t="_VI Default Name (Edit and make value default)", s=w297, f="Name:") -> (s? t:f=w298:string)
            n179 = Bundle By Name(cluster=T4 {"Title"="", "Description"="", "icon image path (.bmp)"=path "", "Help Link"="", "WireThrough Terminal Names"={"WireThrough Top In"="", "WireThrough Bottom In"="", "WireThrough Top Out"="", "WireThrough Bottom Out"=""}, "Instrument Driver Method Descriptor Array"=[]} ("Scripter Input"), "Instrument Driver Method Descriptor Array"=w294, "WireThrough Terminal Names"="_WireThrough Info (Edit and make value default)", "Title"=w298, "Description"="" ("Title")) -> (→"_Scripter Input":T4)
            n180 = Build Array(w282) -> (→"_Connection Informations":T17)
          }
        }
      }
      n181 = Unregister For Events(event registration refnum=w144) -> ()  [unwired: 1 in, 1 out]
    }
  }
  "_create Callback?" <- FALSE ("_create Callback?")
